vi "Reset Acyclic Channels.vi"(8 "error in (no error)":errorcluster, 11 "reference in":refnum<class "VeriStandTestCase.lvclass">) -> (0 "error out":errorcluster, 3 "reference out":refnum<class "VeriStandTestCase.lvclass">)   [LabVIEW 2020]
uses:
  1e32ca70-98be-4c49-9a55-e48adc1a34b6.vi
  <vilib>/NI VeriStand/Execution/Workspace/NI VeriStand - Set Multiple Channel Values.vi
  niveristand-custom-device-testing-tools/VeriStandTestUtilities/VeriStandTestUtilities.lvlib
  <vilib>/NI VeriStand/Execution/Workspace/NI_VS Workspace ExecutionAPI.lvlib
  niveristand-custom-device-testing-tools/VeriStandTestCase/VeriStandTestCase.lvclass
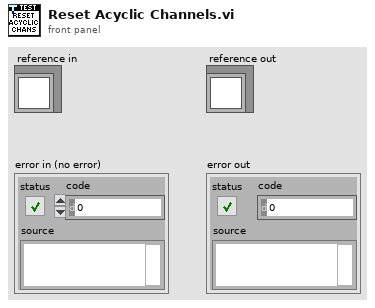
[diagram p1: front panel]
types:
  T1 = typedef "NI_VS Workspace ExecutionAPI.lvlib/WorkspaceAPI.ctl" = refnum<k24>
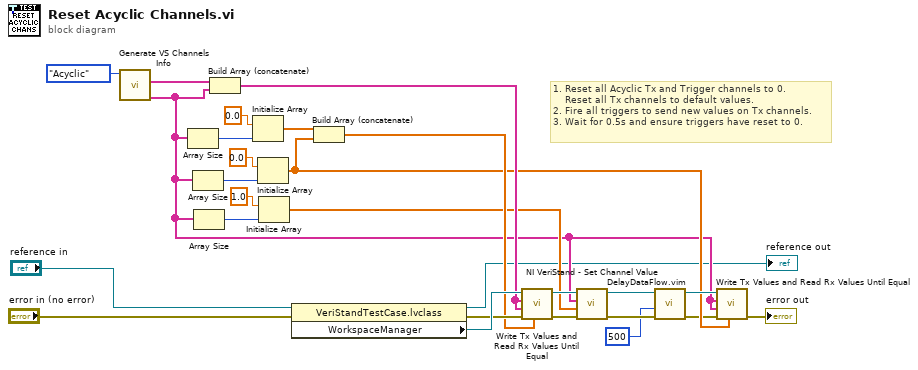
[diagram p0: block diagram]
diagram:
  # "1. Reset all Acyclic Tx and Trigger channels to 0.\n    Reset all Tx channels to default values.\n2. Fire all triggers to send new values on Tx channels.\n3. Wait for 0.5s and ensure triggers have reset to 0."
  n1 = call "Generate VS Channels Info.vi"("Transfer Type"=enum16{"Acyclic", "Scheduled"}."Acyclic") -> ("Tx Trigger Channels Array"=w3:string[], "Tx Channels Array"=w24:string[])  [unwired: 6 in, 3 out]
  n2 = Array Size(array=w3) -> (size(s)=w5:i32)
  n3 = Array Size(array=w3) -> (size(s)=w23:i32)
  n4 = Array Size(array=w3) -> (size(s)=w14:i32)
  n5 = Build Array (concatenate)(w24, w3) -> (w20:string[])
  n6 = Initialize Array(0.0 ("element"), w5) -> (w4:dbl[])
  n7 = Initialize Array(0.0 ("element"), w23) -> (w11:dbl[])
  n8 = Initialize Array(1.0 ("element"), w14) -> (w12:dbl[])
  n9 = property class="VeriStandTestCase.lvclass"(reference="reference in", error in="error in (no error)") -> (reference out=→"reference out":refnum<class "VeriStandTestCase.lvclass">, error out=w21:errorcluster, "WorkspaceManager"=w25:T1)
  n10 = Build Array (concatenate)(w4, w11) -> (w19:dbl[])
  n11 = call "Write Tx Values and Read Rx Values Until Equal.vi"("Tx values"=w19, "error in"=w21, "Rx aliases"=w20, "Tx aliases"=w20, "workspace manager in"=w25) -> ("error out"=w18:errorcluster, "workspace manager out"=w17:T1)  [unwired: 4 in, 1 out]
  n12 = call-poly <vilib>:"NI VeriStand - Set Channel Value.vi"("error in (no error)"=w18, "Values"=w12, "Channels"=w3, "WorkspaceManager in"=w17) -> ("error out"=w16:errorcluster, "WorkspaceManager out"=w15:T1)  [unwired: 6 in]
  n13 = call "DelayDataFlow.vim"("value in"=w16, "milliseconds to wait"=u32 500) -> ("value out"=w10:errorcluster)  [unwired: 2 in, 1 out]
  n14 = call "Write Tx Values and Read Rx Values Until Equal.vi"("Tx values"=w11, "error in"=w10, "Rx aliases"=w3, "Tx aliases"=w3, "workspace manager in"=w15) -> ("error out"=→"error out":errorcluster)  [unwired: 4 in, 2 out]
